vi "Score and Rank Objects.vi"(6 "Targets":i32=3, 8 "Annotations":enum16{"None", "Good", "All"}(ring)=enum."Good", 9 "Score Limit":dbl=70.0, 10 "Object Info":T3(array[cluster]), 11 "Image in":T2) -> (0 "Object Info":T1(array[cluster]), 3 "Annotated Image":T2)   [LabVIEW 2015]
doc: "Use the location, size, and other factors to score and rank the objects. Optionally show annotations over the objects."
uses:
  <vilib>/vision/Image Controls.llb/IMAQ Image.ctl
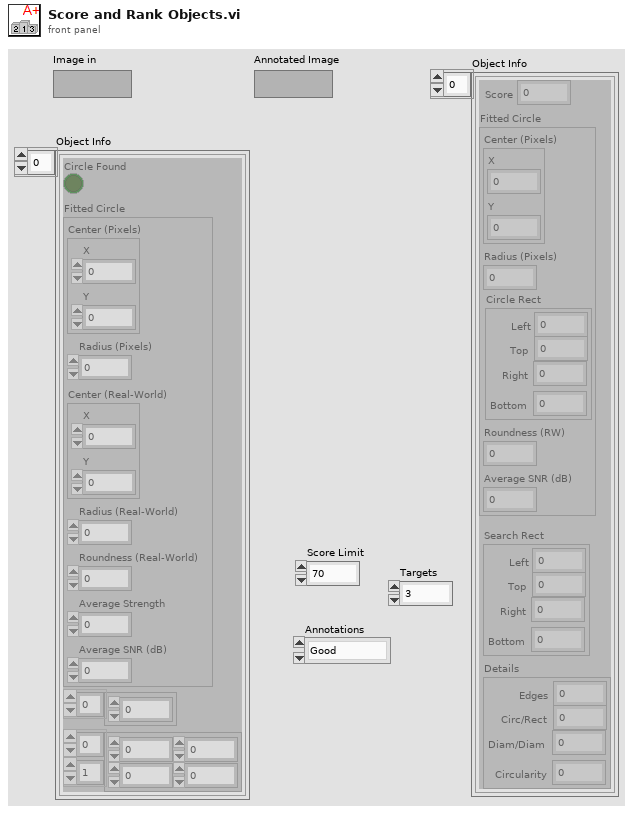
[diagram p1: front panel]
types:
  T1 = cluster{"Score":dbl, "Fitted Circle":cluster{"Center (Pixels)":cluster{"X":sgl, "Y":sgl}, "Radius (Pixels)":dbl, "Circle Rect":cluster{"Left":sgl, "Top":sgl, "Right":sgl, "Bottom":sgl}, "Roundness (RW)":dbl, "Average SNR (dB)":dbl}, "Search Rect":cluster{"Left":sgl, "Top":sgl, "Right":sgl, "Bottom":sgl}, "Details":cluster{"Edges":sgl, "Circ/Rect":sgl, "Diam/Diam":sgl, "Circularity":sgl}}[]
  T2 = typedef "IMAQ Image.ctl" = refnum<image>
  T3 = cluster{"Circle Found":bool, "Fitted Circle":cluster{"Center (Pixels)":cluster{"X":sgl, "Y":sgl}, "Radius (Pixels)":dbl, "Center (Real-World)":cluster{"X":sgl, "Y":sgl}, "Radius (Real-World)":dbl, "Roundness (Real-World)":dbl, "Average Strength":dbl, "Average SNR (dB)":dbl}, dbl[], dbl[][]}[]
  T4 = cluster{"Score":dbl, "Fitted Circle":cluster{"Center (Pixels)":cluster{"X":sgl, "Y":sgl}, "Radius (Pixels)":dbl, "Rect":cluster{"Left":sgl, "Top":sgl, "Right":sgl, "Bottom":sgl}, "Roundness (RW)":dbl, "Average SNR (dB)":dbl}, "Rect":cluster{"Left":sgl, "Top":sgl, "Right":sgl, "Bottom":sgl}, "Details":cluster{"Edges":sgl, "Circ/Rect":sgl, "Diam/Diam":sgl, "Circularity":sgl}}[]
  T5 = cluster{"Desired Font (Application)":enum16{"User-specified Font", "Application Font", "System Font", "Dialog Font"}, "[User-specified Font]":cluster{"Font Name":string, "Size":i16, "Strikeout?":bool, "Italic?":bool, "Underline?":bool, "Outline?":bool, "Shadow?":bool, "Bold?":bool, "Rotation Angle":dbl}, "Horizontal Alignment":i16, "Vertical Alignment":i16}
  T6 = cluster{"Center (Pixels)":cluster{"X":sgl, "Y":sgl}, "Radius (Pixels)":dbl, "Circle Rect":cluster{"Left":sgl, "Top":sgl, "Right":sgl, "Bottom":sgl}, "Roundness (RW)":dbl, "Average SNR (dB)":dbl}
  T7 = cluster{"Left":sgl, "Top":sgl, "Right":sgl, "Bottom":sgl}
  T8 = cluster{"Edges":sgl, "Circ/Rect":sgl, "Diam/Diam":sgl, "Circularity":sgl}
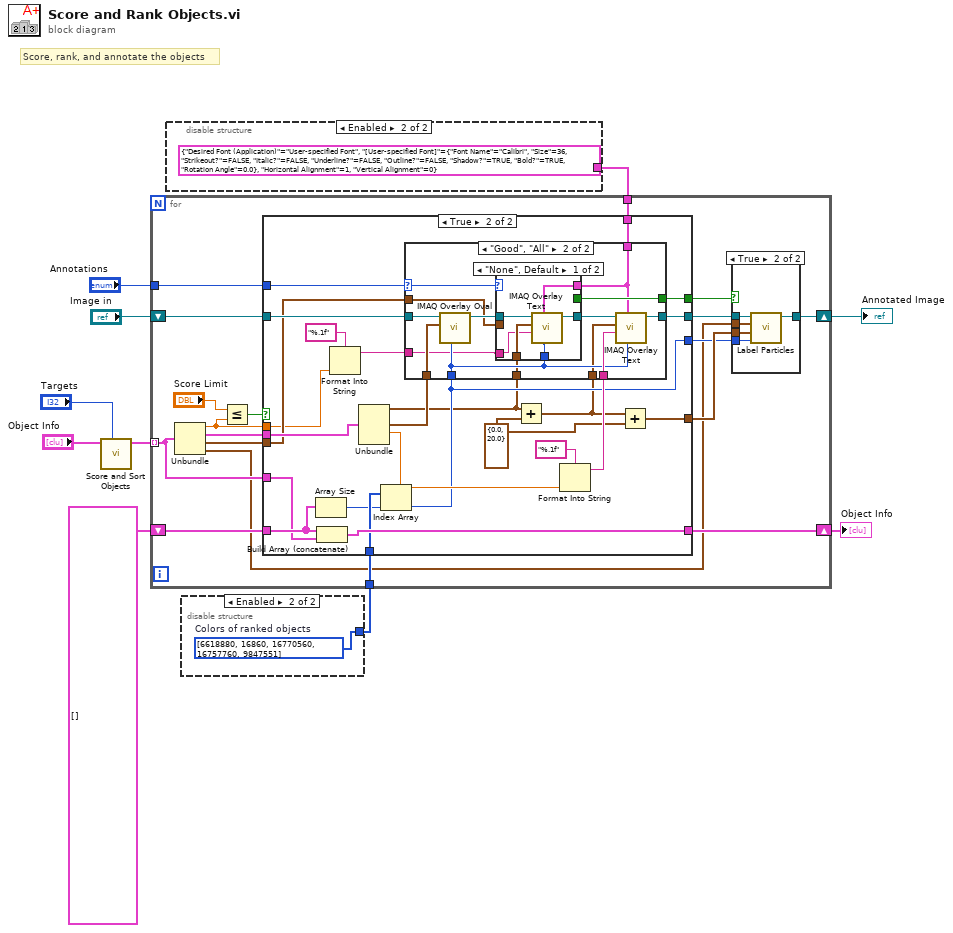
[diagram p0: block diagram]
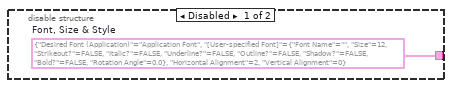
[diagram p2: hidden frame]
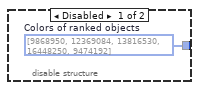
[diagram p3: hidden frame]
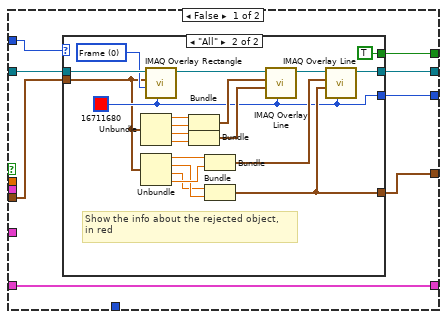
[diagram p5: hidden frame]
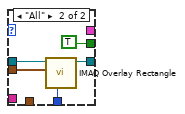
[diagram p8: hidden frame]
diagram:
  # "Score, rank, and annotate the objects"
  n1 = call "Score and Sort Objects.vi"("Targets"="Targets", "Object Info"="Object Info") -> ("Object Info"=w5:T1)  [unwired: 9 in]
  n2 = disable-structure shown="Enabled" {
    disable-tunnel: [w11 T5 {"Desired Font (Application)"=enum."User-specified Font", "[User-specified Font]"={"Font Name"="Calibri", "Size"=36, "Strikeout?"=FALSE, "Italic?"=FALSE, "Underline?"=FALSE, "Outline?"=FALSE, "Shadow?"=TRUE, "Bold?"=TRUE, "Rotation Angle"=0.0}, "Horizontal Alignment"=1, "Vertical Alignment"=0} ("Font, Size & Style 2")] -> w1
    frame Disabled {
      w11 = T5 {"Desired Font (Application)"=enum."Application Font", "[User-specified Font]"={"Font Name"="", "Size"=12, "Strikeout?"=FALSE, "Italic?"=FALSE, "Underline?"=FALSE, "Outline?"=FALSE, "Shadow?"=FALSE, "Bold?"=FALSE, "Rotation Angle"=0.0}, "Horizontal Alignment"=2, "Vertical Alignment"=0}  # Font, Size & Style
    }
    frame Enabled {
    }
  }
  n3 = disable-structure shown="Enabled" {
    disable-tunnel: [w13 w14] -> w8
    frame Disabled {
      w13 = u32[] [9868950, 12369084, 13816530, 16448250, 9474192]  # Colors of ranked objects
    }
    frame Enabled {
      w14 = u32[] [6618880, 16860, 16770560, 16757760, 9847551]  # Colors of ranked objects
    }
  }
  n4 = for {
    tunnel: w5 -> [w19] mode=indexing
    shift-right: [w30] -> w9
    shift-left: "Image in" -> [w29]
    shift-right: [w28] -> w4
    shift-left: T4 [] ("Object Info") -> [w27]
    tunnel: w1 -> [w26]
    tunnel: w8 -> [w25]
    tunnel: "Annotations" -> [w21]
    n5 = Unbundle(w19) -> ("Score"=w16:dbl, "Fitted Circle"=w31:T6, "Search Rect"=w32:T7, "Details"=w15:T8)
    n6 = Less Or Equal?(x="Score Limit", y=w16) -> (x <= y?=w17:bool)
    n7 = case shown="True" w17 {
      tunnel: w31 -> [_ w81]
      tunnel: w29 -> [w46 w91]
      tunnel: [w40 w90] -> w28
      tunnel: w32 -> [w45 w78]
      tunnel: [w44 w89] -> w24
      tunnel: w26 -> [_ w84]
      tunnel: w25 -> [_ w86]
      tunnel: [w43 w83] -> w23
      tunnel: w21 -> [w42 w76]
      tunnel: [w41 w77] -> w22
      tunnel: w27 -> [w40 w82]
      tunnel: [w39 w75] -> w20
      tunnel: w19 -> [_ w74]
      tunnel: w16 -> [_ w68]
      frame False {
        n8 = case shown="\"All\"" w42 {
          tunnel: w46 -> [w47 w67]
          tunnel: w45 -> [_ w49]
          tunnel: [w47 w52] -> w44
          tunnel: [_ w51] -> w43
          tunnel: [_ w50] -> w41
          tunnel: [_ TRUE] -> w39
          frame "None", Default {
            # "Rejected, not supposed to annotate"
          }
          frame "All" {
            w54 = u32 0 items=["Frame", "Fill", "Highlight"] ("Drawing Mode (Frame)")
            w50 = u32 16711680 ("Color")
            # "Show the info about the rejected object,\nin red"
            n9 = Unbundle(w49) -> ("Left"=w64:sgl, "Top"=w63:sgl, "Right"=w62:sgl, "Bottom"=w61:sgl)
            n10 = Unbundle(w49) -> ("Left"=w60:sgl, "Top"=w58:sgl, "Right"=w57:sgl, "Bottom"=w59:sgl)
            n11 = call "IMAQ Overlay Rectangle"("Color"=w50, "Drawing Mode (Frame)"=w54, "Rectangle"=w49, "Image"=w67) -> ("Image Out"=w66:T2)  [unwired: 6 in, 1 out]
            n12 = Bundle("Left"=w64, "Top"=w63) -> (w53:cluster{"Left":sgl, "Top":sgl})  [unwired: 1 in]
            n13 = Bundle("Right"=w62, "Bottom"=w61) -> (w56:cluster{"Right":sgl, "Bottom":sgl})  [unwired: 1 in]
            n14 = Bundle("Left"=w60, "Bottom"=w59) -> (w55:cluster{"Left":sgl, "Bottom":sgl})  [unwired: 1 in]
            n15 = Bundle("Right"=w57, "Top"=w58) -> (w51:cluster{"Right":sgl, "Top":sgl})  [unwired: 1 in]
            n16 = call "IMAQ Overlay Line"("Color"=w50, "End Point"=w56, "Start Point"=w53, "Image"=w66) -> ("Image Out"=w65:T2)  [unwired: 6 in, 1 out]
            n17 = call "IMAQ Overlay Line"("Color"=w50, "End Point"=w51, "Start Point"=w55, "Image"=w65) -> ("Image Out"=w52:T2)  [unwired: 6 in, 1 out]
          }
        }
      }
      frame True {
        w69 = cluster{dbl, dbl} {0.0, 20.0} ("x+y")
        n18 = Array Size(array=w82) -> (size(s)=w85:i32)
        n19 = Build Array (concatenate)(w82, w74) -> (w90:T1)
        n20 = Format Into String(format string="%.1f", w68) -> (resulting string=w72:string)  [unwired: 2 in, 1 out]
        n21 = Unbundle(w81) -> ("Center (Pixels)"=w70:cluster{"X":sgl, "Y":sgl}, "Circle Rect"=w80:T7, "Roundness (RW)"=w79:dbl)  [unwired: 2 out]
        n22 = Index Array(array=w86, index=w85) -> (element=w77:u32)
        n23 = Add(x=w70, y=w69) -> (x+y=w71:cluster{dbl, dbl})
        n24 = Format Into String(format string="%.1f", w79) -> (resulting string=w87:string)  [unwired: 2 in, 1 out]
        n25 = case shown="\"Good\", \"All\"" w76 {
          selector: w76 -> [_ w97]
          tunnel: w91 -> [w92 w106]
          tunnel: [w92 w104] -> w89
          tunnel: w87 -> [_ w103]
          tunnel: w84 -> [_ w95]
          tunnel: w77 -> [_ w101]
          tunnel: w71 -> [_ w100]
          tunnel: w80 -> [_ w99]
          tunnel: w78 -> [_ w98]
          tunnel: [_ w96] -> w75
          tunnel: w70 -> [_ w94]
          tunnel: w72 -> [_ w93]
          frame "None", Default {
          }
          frame "Good", "All" {
            n26 = call "IMAQ Overlay Oval"("Color"=w101, "Bounding Rectangle"=w99, "Image"=w106) -> ("Image Out"=w105:T2)  [unwired: 7 in, 1 out]
            n27 = case shown="\"None\", Default" w97 {
              tunnel: w98 -> [_ w117]
              tunnel: w105 -> [w112 w116]
              tunnel: [w111 w115] -> w102
              tunnel: w101 -> [w110 w114]
              tunnel: [_ TRUE] -> w96
              tunnel: w95 -> [w109 _]
              tunnel: w94 -> [w108 _]
              tunnel: w93 -> [w107 _]
              frame "None", Default {
                n28 = call "IMAQ Overlay Text"("Text Color (black)"=w110, "Font, Size & Style"=w109, "String"=w107, "Origin"=w108, "Image"=w112) -> ("Image Out"=w111:T2)  [unwired: 5 in, 1 out]
              }
              frame "All" {
                n29 = call "IMAQ Overlay Rectangle"("Color"=w114, "Rectangle"=w117, "Image"=w116) -> ("Image Out"=w115:T2)  [unwired: 7 in, 1 out]
              }
            }
            n30 = call "IMAQ Overlay Text"("Text Color (black)"=w101, "Font, Size & Style"=w95, "String"=w103, "Origin"=w100, "Image"=w102) -> ("Image Out"=w104:T2)  [unwired: 5 in, 1 out]
          }
        }
        n31 = Add(x=w71, y=w69) -> (x+y=w83:cluster{dbl, dbl})
      }
    }
    n32 = case shown="True" w20 {
      tunnel: [w33 w38] -> w30
      tunnel: w24 -> [w33 w37]
      tunnel: w23 -> [_ w36]
      tunnel: w22 -> [_ w35]
      tunnel: w15 -> [_ w34]
      frame False {
      }
      frame True {
        n33 = call "Label Particles.vi"("Color"=w35, "Location"=w36, "Details"=w34, "Image"=w37) -> ("Image 2"=w38:T2)  [unwired: 7 in]
      }
    }
  }
  "Annotated Image" <- w9
  "Object Info" <- w4
